vi "PSDEV_Device Save Config To IniFile.vi"(8 "error in":errorcluster caption="错误输入（无错误）", 11 "Card":T1={"Module Type"="", "Module Name"="", "ModuSN"="", "ModuIP"="", "Used?"=FALSE, "Connected"=FALSE, "Timing*"={"Sample Rate"=1000.0}, "Channels"=[]}) -> (0 "error out":errorcluster caption="错误输出")   [LabVIEW 2016]
uses:
  <vilib>/Utility/config.llb/NI_LVConfig.lvlib
  <vilib>/Utility/config.llb/Write Key (Boolean).vi
  <vilib>/Utility/config.llb/Write Key (I32).vi
  <vilib>/Utility/config.llb/Write Key (U32).vi
  <vilib>/Utility/config.llb/Write Key (Double).vi
  <vilib>/Utility/config.llb/Write Key (String).vi
  DAQ-Config/Controls/PSCHN_Channel Para.ctl
  DAQ-Config/Controls/PSCHN_Card Para.ctl
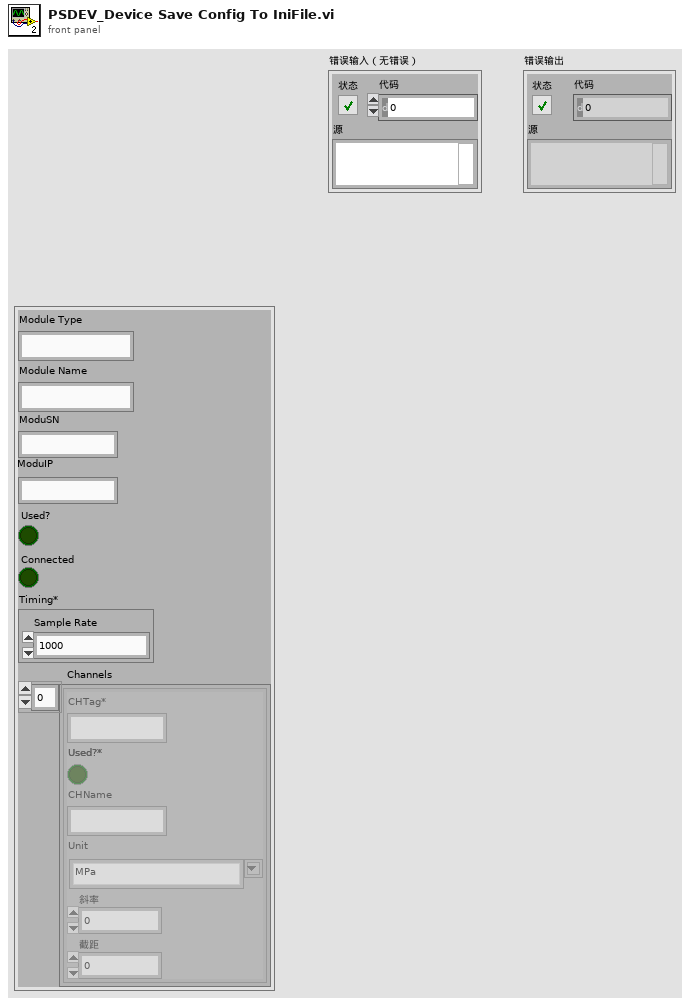
[diagram p1: front panel]
types:
  T1 = typedef "PSCHN_Card Para.ctl" = cluster{"Module Type":string, "Module Name":string, "ModuSN":string, "ModuIP":string, "Used?":bool, "Connected":bool, "Timing*":cluster{"Sample Rate":dbl}, "Channels":T2[]}
  T2 = typedef "PSCHN_Channel Para.ctl" = cluster{"CHTag*":string, "Used?*":bool, "CHName":string, "Unit":string, "斜率":dbl, "截距":dbl}
  T3 = cluster{"TREE PNG":path, "User Guide":path, "DefaultSave":path, "BuildPath":path, "Image":path, "Modules":path, "Configuration":path, "License":path, "SplitFiles":path, "System.ini":path}
  T4 = typedef "NI_LVConfig.lvlib/Config Data RefNum.ctl" = refnum<k1>
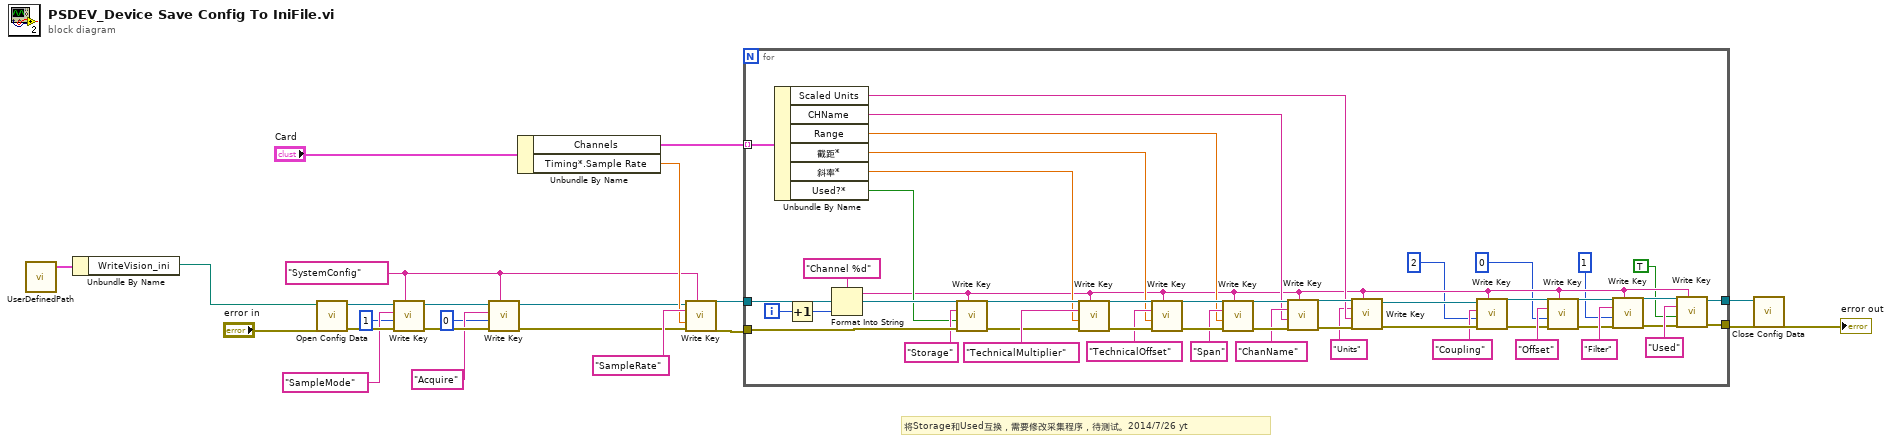
[diagram p0: block diagram]
diagram:
  w8 = "SystemConfig" ("section")
  # "将Storage和Used互换，需要修改采集程序，待测试。2014/7/26 yt"
  n1 = call "UserDefinedPath.vi"() -> ("UserDefinedPath"=w2:T3)  [unwired: 11 in]
  n2 = Unbundle By Name(w2) -> ("WriteVision_ini"=w1:path)
  n3 = call <vilib>:"Open Config Data.vi"("error in (no error)"="error in", "configuration file path"=w1) -> ("error out"=w13:errorcluster, "refnum"=w14:T4)  [unwired: 7 in, 1 out]
  n4 = call-poly <vilib>:"Write Key.vi"("section"=w8, "error in (no error)"=w13, "value"=u32 1, "key"="SampleMode", "refnum"=w14) -> ("error out"=w12:errorcluster, "refnum out"=w10:T4)  [unwired: 4 in, 1 out]
  n5 = call-poly <vilib>:"Write Key.vi"("section"=w8, "error in (no error)"=w12, "value"=u32 0, "key"="Acquire", "refnum"=w10) -> ("error out"=w11:errorcluster, "refnum out"=w9:T4)  [unwired: 4 in, 1 out]
  n6 = Unbundle By Name("Card") -> ("Channels"=w20:T2[], "Timing*.Sample Rate"=w17:dbl)
  n7 = call-poly <vilib>:"Write Key.vi"("section"=w8, "error in (no error)"=w11, "value"=w17, "key"="SampleRate", "refnum"=w9) -> ("error out"=w22:errorcluster, "refnum out"=w19:T4)  [unwired: 4 in, 1 out]
  n8 = for {
    tunnel: w22 -> [w51]
    tunnel: [w33] -> w21
    tunnel: w20 -> [w70] mode=indexing
    tunnel: w19 -> [w53]
    tunnel: [w25] -> w18
    i -> [w69]
    n9 = Unbundle By Name(w70) -> ("Scaled Units"=w59:string, "CHName"=w44:string, "Range"=w45:dbl, "截距*"=w46:dbl, "斜率*"=w47:dbl, "Used?*"=w48:bool)
    n10 = Increment(x=w69) -> (x+1=w24:i32)
    n11 = Format Into String(format string="Channel %d" ("格式字符串"), w24) -> (resulting string=w32:string)  [unwired: 2 in, 1 out]
    n12 = call-poly <vilib>:"Write Key.vi"("section"=w32, "error in (no error)"=w51, "value"=w48, "key"="Storage", "refnum"=w53) -> ("error out"=w50:errorcluster, "refnum out"=w52:T4)  [unwired: 4 in, 1 out]
    n13 = call-poly <vilib>:"Write Key.vi"("section"=w32, "error in (no error)"=w50, "value"=w47, "key"="TechnicalMultiplier", "refnum"=w52) -> ("error out"=w67:errorcluster, "refnum out"=w63:T4)  [unwired: 4 in, 1 out]
    n14 = call-poly <vilib>:"Write Key.vi"("section"=w32, "error in (no error)"=w67, "value"=w46, "key"="TechnicalOffset", "refnum"=w63) -> ("error out"=w66:errorcluster, "refnum out"=w62:T4)  [unwired: 4 in, 1 out]
    n15 = call-poly <vilib>:"Write Key.vi"("section"=w32, "error in (no error)"=w66, "value"=w45, "key"="Span", "refnum"=w62) -> ("error out"=w65:errorcluster, "refnum out"=w61:T4)  [unwired: 4 in, 1 out]
    n16 = call-poly <vilib>:"Write Key.vi"("section"=w32, "error in (no error)"=w65, "value"=w44, "key"="ChanName", "refnum"=w61) -> ("error out"=w64:errorcluster, "refnum out"=w60:T4)  [unwired: 4 in, 1 out]
    n17 = call-poly <vilib>:"Write Key.vi"("section"=w32, "error in (no error)"=w64, "value"=w59, "key"="Units", "refnum"=w60) -> ("error out"=w34:errorcluster, "refnum out"=w30:T4)  [unwired: 4 in, 1 out]
    n18 = call-poly <vilib>:"Write Key.vi"("section"=w32, "error in (no error)"=w34, "value"=2, "key"="Coupling", "refnum"=w30) -> ("error out"=w35:errorcluster, "refnum out"=w38:T4)  [unwired: 4 in, 1 out]
    n19 = call-poly <vilib>:"Write Key.vi"("section"=w32, "error in (no error)"=w35, "value"=0, "key"="Offset", "refnum"=w38) -> ("error out"=w36:errorcluster, "refnum out"=w39:T4)  [unwired: 4 in, 1 out]
    n20 = call-poly <vilib>:"Write Key.vi"("section"=w32, "error in (no error)"=w36, "value"=1, "key"="Filter", "refnum"=w39) -> ("error out"=w37:errorcluster, "refnum out"=w40:T4)  [unwired: 4 in, 1 out]
    n21 = call-poly <vilib>:"Write Key.vi"("section"=w32, "error in (no error)"=w37, "value"=TRUE, "key"="Used", "refnum"=w40) -> ("error out"=w33:errorcluster, "refnum out"=w25:T4)  [unwired: 4 in, 1 out]
  }
  n22 = call <vilib>:"Close Config Data.vi"("error in (no error)"=w21, "refnum"=w18) -> ("error out"=→"error out":errorcluster)  [unwired: 8 in, 1 out]
